vi "Open-session.vi"(8 "error in (no error)":errorcluster, 9 "Camport":u32, 10 "Framegrabber board":i32, 11 "Camera in":refnum<class "Camera.lvclass">) -> (0 "error out":errorcluster, 2 "IMAQ Session":refnum<k11>, 3 "Camera out":refnum<class "Camera.lvclass">)   [LabVIEW 2013, in "CameraVision.lvlib" / "Camera.lvclass"]
uses:
  Camera.lvclass
  Camera.lvclass/Camera.ctl
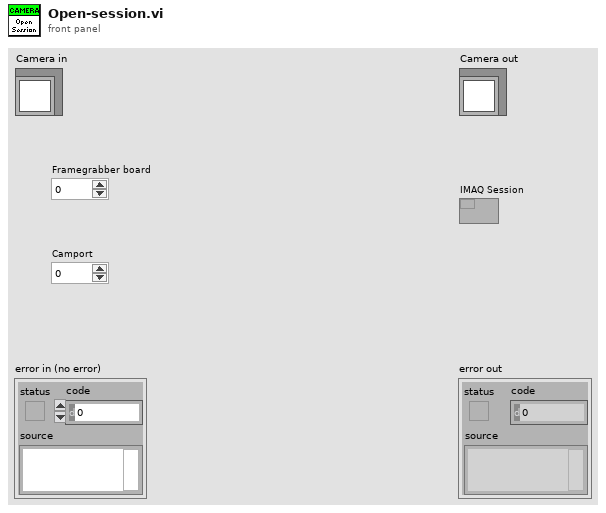
[diagram p1: front panel]
types:
  T1 = cluster{"Max. offset X":u32, "Max. offset Y":u32, "Offset step size X":u32, "Offset step size Y":u32}
  T2 = cluster{"Max. width":u32, "Max. height":u32, "Step size width":dbl, "Min. width":u32, "Min. height":u32, "Step size height":dbl}
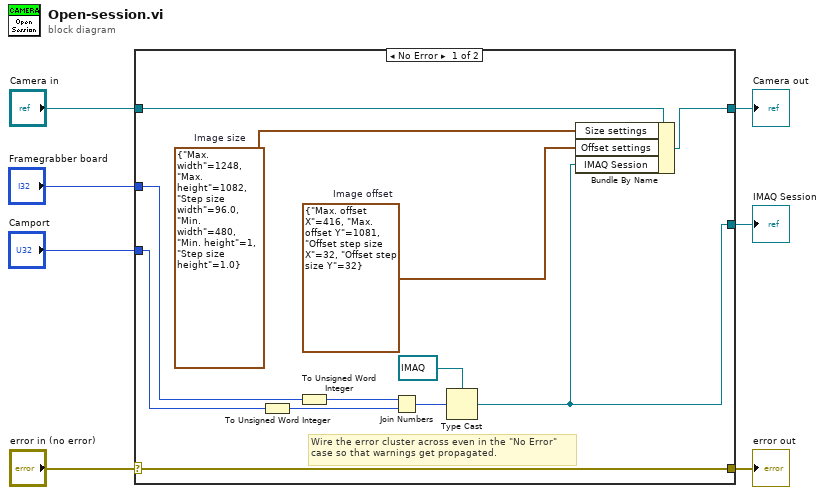
[diagram p0: block diagram]
diagram:
  n1 = case shown="No Error" "error in (no error)" {
    selector: "error in (no error)" -> [w13 w21]
    tunnel: [w13 w21] -> w6
    tunnel: [w14 w20] -> w4
    tunnel: "Camera in" -> [w15 w20]
    tunnel: "Framegrabber board" -> [w17 _]
    tunnel: "Camport" -> [w16 _]
    tunnel: [w10 _] -> w1
    frame No Error {
      w11 = T1 {"Max. offset X"=416, "Max. offset Y"=1081, "Offset step size X"=32, "Offset step size Y"=32}  # Image offset
      w12 = T2 {"Max. width"=1248, "Max. height"=1082, "Step size width"=96.0, "Min. width"=480, "Min. height"=1, "Step size height"=1.0}  # Image size
      # "Wire the error cluster across even in the \"No Error\"\ncase so that warnings get propagated."
      n2 = To Unsigned Word Integer(number=w16) -> (unsigned 16bit integer=w8:u16)
      n3 = To Unsigned Word Integer(number=w17) -> (unsigned 16bit integer=w9:u16)
      n4 = Join Numbers(hi=w9, lo=w8) -> ((hi.lo)=w19:u32)
      n5 = Type Cast(type=refnum<k11> refnum ("IMAQ Session in"), x=w19) -> (*(type *) &x=w10:refnum<k11>)
      n6 = Bundle By Name(cluster=w15, "Size settings"=w12, "Offset settings"=w11, "IMAQ Session"=w10) -> (w14:refnum<class "Camera.lvclass">)
    }
    frame Error {
    }
  }
  "error out" <- w6
  "Camera out" <- w4
  "IMAQ Session" <- w1
